vi "Max Packet Length.vi"() -> (3 "Max Packet Length":i32=254)   [LabVIEW 2015, in "LSR Transmission.lvlib"]
uses:
  LSR Transmission.lvlib
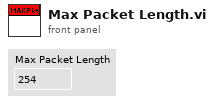
[diagram p1: front panel]
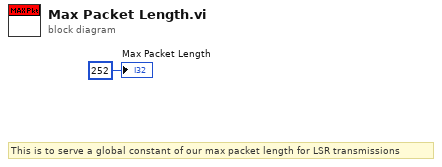
[diagram p0: block diagram]
diagram:
  # "This is to serve a global constant of our max packet length for LSR transmissions"
  "Max Packet Length" <- 252 ("y")
